vi "Configure Current Limit.vi"(7 "Limit (0.0 amps)":dbl format="%^.3e", 8 "error in (no error)":errorcluster {"code" format="%.0x"}, 9 "Behavior (0: Regulatory Limit)":i32(ring) items=["Regulatory Limit", "Trip Limit"], 10 "Channel Name (1)":string="1", 11 "VISA resource name":refnum<visa-resource-name>) -> (0 "error out":errorcluster {"code" format="%.0x"}, 3 "VISA resource name out":refnum<visa-resource-name>)   [LabVIEW 2016, in "Agilent N6700 Series.lvlib"]
doc: "Configures the current limit. You specify the output current limit value and the behavior of the power supply when the output current is greater than or equal to that value."
uses:
  <instrlib>/Agilent N6700 Series/Agilent N6700 Series.lvlib
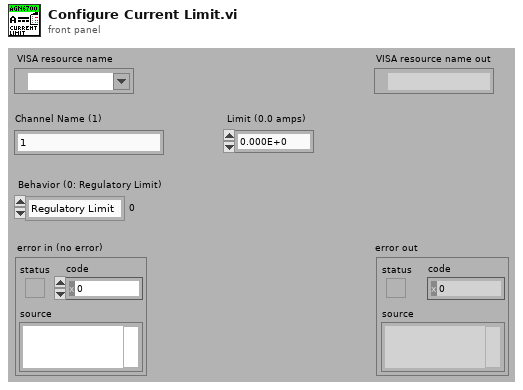
[diagram p1: front panel]
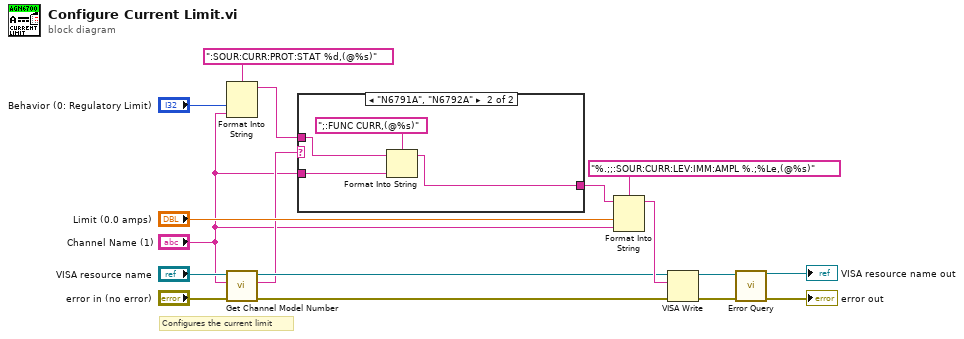
[diagram p0: block diagram]
diagram:
  # "Configures the current limit"
  n1 = Format Into String(format string=":SOUR:CURR:PROT:STAT %d,(@%s)", "Behavior (0: Regulatory Limit)", "Channel Name (1)") -> (resulting string=w3:string)  [unwired: 2 in, 1 out]
  n2 = call <instrlib>:"Get Channel Model Number.vi"("error in (no error)"="error in (no error)", "Channel Name (1)"="Channel Name (1)", "VISA resource name"="VISA resource name") -> ("error out"=w6:errorcluster, "Model Number"=w4:string, "VISA resource name out"=w7:refnum<visa-resource-name>)  [unwired: 6 in]
  n3 = case shown="\"N6791A\", \"N6792A\"" w4 {
    tunnel: w3 -> [w18 w20]
    tunnel: [w18 w22] -> w2
    tunnel: "Channel Name (1)" -> [_ w19]
    frame Default {
      # "Only N679xA need to change priority mode."
    }
    frame "N6791A", "N6792A" {
      n4 = Format Into String(format string=";:FUNC CURR,(@%s)", initial string=w20, w19) -> (resulting string=w22:string)  [unwired: 1 in, 1 out]
    }
  }
  n5 = Format Into String(format string="%.;;:SOUR:CURR:LEV:IMM:AMPL %.;%Le,(@%s)", initial string=w2, "Limit (0.0 amps)", "Channel Name (1)") -> (resulting string=w13:string)  [unwired: 1 in, 1 out]
  n6 = VISA Write(VISA resource name=w7, write buffer=w13, error in (no error)=w6) -> (VISA resource name out=w10:refnum<visa-resource-name>, error out=w9:errorcluster)  [unwired: 1 out]
  n7 = call <instrlib>:"Error Query.vi"("VISA resource name"=w10, "error in (no error)"=w9) -> ("VISA resource name out"=→"VISA resource name out":refnum<visa-resource-name>, "error out"=→"error out":errorcluster)  [unwired: 10 in, 2 out]
